vi "Float To String.vi"(4 "Type Enum [auto]":T1, 5 "Formatting (auto)":string, 6 "Variant":variant, 8 "error in (no error)":errorcluster, 10 "Multiply":variant, 11 "Registry Object":refnum<class "Carya Config.lvclass">) -> (0 "error out":errorcluster, 2 "resulting string":string, 3 "Registry Object":refnum<class "Carya Config.lvclass">)   [LabVIEW 2013, in "Carya Config.lvclass"]
doc: "Copyright 2018, Carya Automatisering, Wiebe Walstra."
uses:
  Carya Config.lvclass
  <vilib>/Utility/VariantDataType/Type.ctl
  <vilib>/Utility/error.llb/Error Cluster From Error Code.vi
  <vilib>/ErrorRing/Error Ring.xnode
  CConfig Variant Accessor/CConfig Variant Accessor.lvclass
  <vilib>/Utility/VariantDataType/VariantType.lvlib
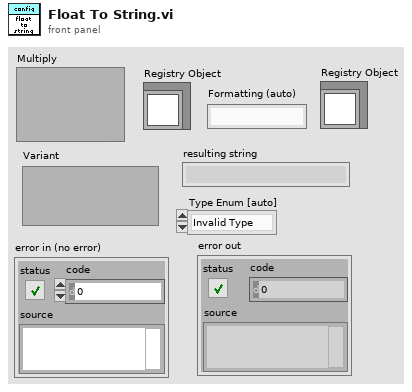
[diagram p1: front panel]
types:
  T1 = typedef "VariantType.lvlib/Type.ctl" = enum8{"Invalid Type", "Void", "I8", "I16", "I32", "I64", "U8", "U16", "U32", "U64", "Single Float", "Double Float", "Extended Float", "Single Complex", "Double Complex", "Extended Complex", "Enum U8", "Enum U16", "Enum U32", "Enum U64", "Single Float With Unit", "Double Float With Unit", "Extended Float With Unit", "Single Complex with Unit", "Double Complex with Unit", "Extended Complex with Unit", "Boolean", "String", "Path", "Picture", "Tag", "Array", "Cluster", "Variant", "LV Variant", "Waveform", "Timestamp", "Digital Waveform", "Digital Data", "ExpressData", "Refnum", "External Data", "VI", "Poly VI", "LabVIEW Class Instance", "Fixed Point"}
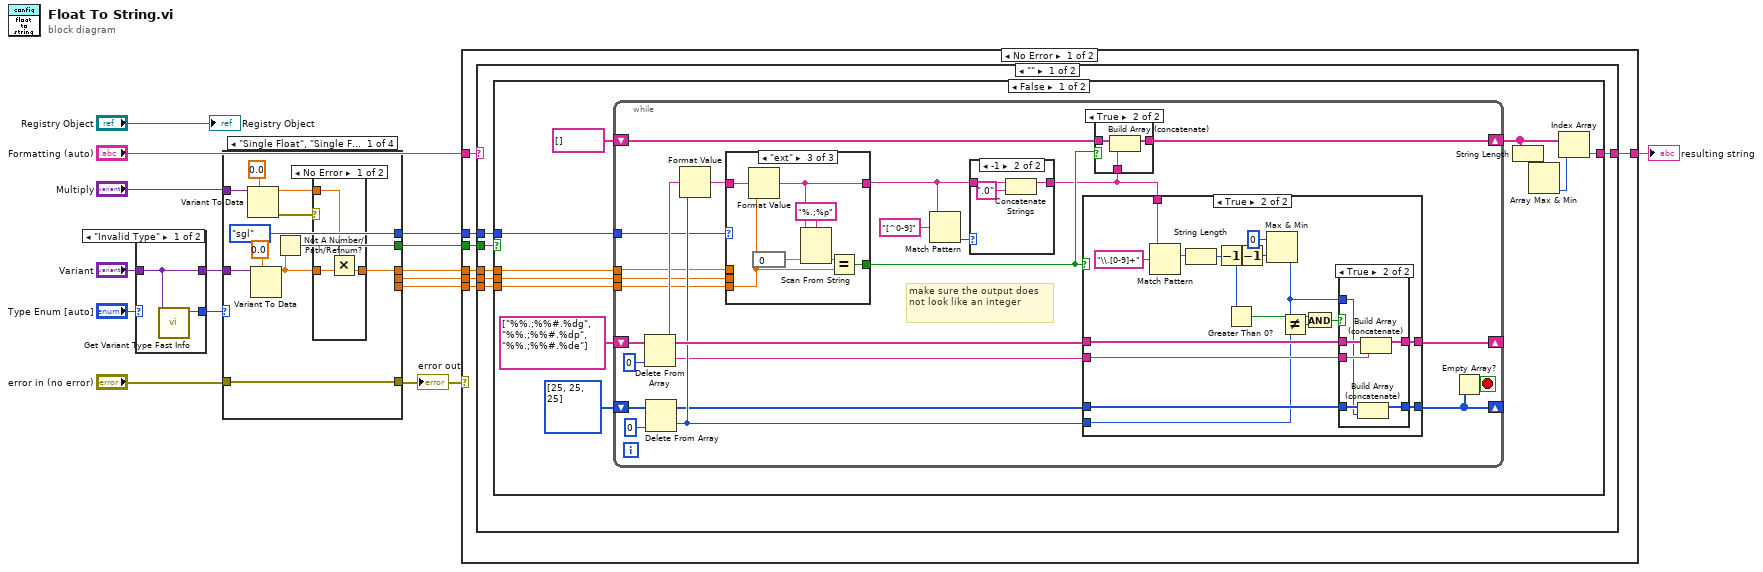
[diagram p0: block diagram]
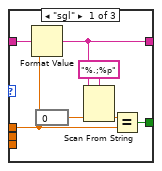
[diagram p3: hidden frame]
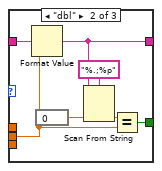
[diagram p4: hidden frame]
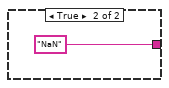
[diagram p8: hidden frame]
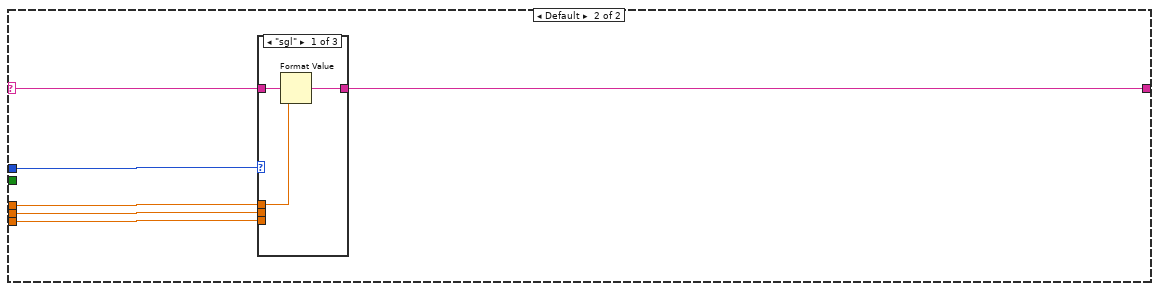
[diagram p9: hidden frame]
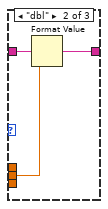
[diagram p10: hidden frame]
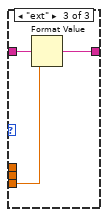
[diagram p11: hidden frame]
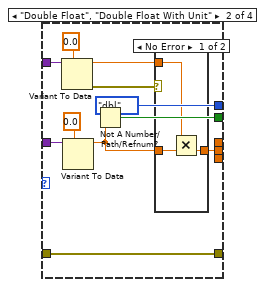
[diagram p15: hidden frame]
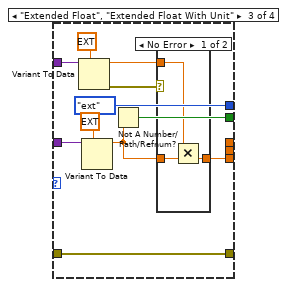
[diagram p17: hidden frame]
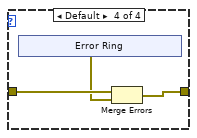
[diagram p19: hidden frame]
diagram:
  n1 = case shown="\"Invalid Type\"" "Type Enum [auto]" {
    selector: "Type Enum [auto]" -> [_ w19]
    tunnel: "Variant" -> [w16 w18]
    tunnel: [w17 w19] -> w5
    tunnel: [w16 w18] -> w7
    frame "Invalid Type" {
      n2 = call "Get Variant Type Fast Info.vi"("Variant"=w16) -> ("Type Enum"=w17:T1)  [unwired: 6 in, 4 out]
    }
    frame Default {
    }
  }
  n3 = case shown="\"Single Float\", \"Single Float With Unit\"" w5 {
    tunnel: [w22 _ _ _] -> w1
    tunnel: [w30 w45 w60 _] -> w13
    tunnel: [_ _ w50 _] -> w12
    tunnel: [_ w35 _ _] -> w11
    tunnel: w7 -> [w28 w43 w58 _]
    tunnel: [enum16{"sgl", "dbl", "ext"}."sgl" ("Type [dbl]") enum16{"sgl", "dbl", "ext"}."dbl" ("Type [dbl]") enum16{"sgl", "dbl", "ext"}."ext" ("Type [dbl]") _] -> w6
    tunnel: "error in (no error)" -> [w26 w41 w56 w67]
    tunnel: [w26 w41 w56 w65] -> w3
    tunnel: "Multiply" -> [w24 w39 w54 _]
    frame "Single Float", "Single Float With Unit" {
      n4 = Variant To Data(type=sgl 0.0, Variant=w24) -> (data=w21:sgl, error out=w20:errorcluster)  [unwired: 1 in]
      n5 = Variant To Data(type=sgl 0.0, Variant=w28) -> (data=w23:sgl)  [unwired: 1 in, 1 out]
      n6 = Not A Number/Path/Refnum?(number/path/refnum=w23) -> (NaN/Path/Refnum?=w30:bool)
      n7 = case shown="No Error" w20 {
        tunnel: w23 -> [w33 w34]
        tunnel: [w32 w34] -> w22
        tunnel: w21 -> [w31 _]
        frame No Error {
          n8 = Multiply(x=w31, y=w33) -> (x*y=w32:sgl)
        }
        frame Error {
        }
      }
    }
    frame "Double Float", "Double Float With Unit" {
      n9 = Variant To Data(type=0.0, Variant=w39) -> (data=w37:dbl, error out=w38:errorcluster)  [unwired: 1 in]
      n10 = Variant To Data(type=0.0, Variant=w43) -> (data=w36:dbl)  [unwired: 1 in, 1 out]
      n11 = Not A Number/Path/Refnum?(number/path/refnum=w36) -> (NaN/Path/Refnum?=w45:bool)
      n12 = case shown="No Error" w38 {
        tunnel: w36 -> [w48 w49]
        tunnel: [w47 w49] -> w35
        tunnel: w37 -> [w46 _]
        frame No Error {
          n13 = Multiply(x=w46, y=w48) -> (x*y=w47:dbl)
        }
        frame Error {
        }
      }
    }
    frame "Extended Float", "Extended Float With Unit" {
      n14 = Variant To Data(type=ext 0.0, Variant=w54) -> (data=w53:ext, error out=w52:errorcluster)  [unwired: 1 in]
      n15 = Variant To Data(type=ext 0.0, Variant=w58) -> (data=w51:ext)  [unwired: 1 in, 1 out]
      n16 = Not A Number/Path/Refnum?(number/path/refnum=w51) -> (NaN/Path/Refnum?=w60:bool)
      n17 = case shown="No Error" w52 {
        tunnel: w51 -> [w63 w64]
        tunnel: [w62 w64] -> w50
        tunnel: w53 -> [w61 _]
        frame No Error {
          n18 = Multiply(x=w61, y=w63) -> (x*y=w62:ext)
        }
        frame Error {
        }
      }
    }
    frame Default {
      n19 = xnode "Error Ring"() -> ("error out"=w66:errorcluster)
      n20 = Merge Errors(w67, w66) -> (w65:errorcluster)
    }
  }
  "error out" <- w3
  n21 = case shown="No Error" w3 {
    tunnel: [w79 _] -> w15
    tunnel: w1 -> [w78 _]
    tunnel: w13 -> [w77 _]
    tunnel: w12 -> [w76 _]
    tunnel: w11 -> [w75 _]
    tunnel: "Formatting (auto)" -> [w74 _]
    tunnel: w6 -> [w73 _]
    frame No Error {
      n22 = case shown="\"\"" w74 {
        selector: w74 -> [_ w178]
        tunnel: [w85 w177] -> w79
        tunnel: w78 -> [w84 w182]
        tunnel: w77 -> [w83 _]
        tunnel: w76 -> [w82 w181]
        tunnel: w75 -> [w81 w180]
        tunnel: w73 -> [w80 w179]
        frame "" {
          n23 = case shown="False" w83 {
            tunnel: [w94 "NaN" ("output string")] -> w85
            tunnel: w84 -> [w90 _]
            tunnel: w82 -> [w88 _]
            tunnel: w81 -> [w87 _]
            tunnel: w80 -> [w86 _]
            frame False {
              n24 = while {
                tunnel: w90 -> [w104]
                shift-right: [w117] -> w92
                shift-left: string[] [] -> [w118]
                shift-right: [w109] -> _
                shift-left: string[] ["%%.;%%#.%dg", "%%.;%%#.%dp", "%%.;%%#.%de"] -> [w116]
                shift-right: [w106] -> _
                shift-left: i32[] [25, 25, 25] -> [w115]
                tunnel: w88 -> [w102]
                tunnel: w87 -> [w103]
                tunnel: w86 -> [w101]
                stop <- w105 stop-if-true
                # "make sure the output does not look like an integer"
                n25 = Delete From Array(array=w116, index=0) -> (deleted portion=w108:string, array with subset deleted=w111:string[])  [unwired: 1 in]
                n26 = Delete From Array(array=w115, index=0) -> (deleted portion=w110:i32, array with subset deleted=w107:i32[])  [unwired: 1 in]
                n27 = Format Value(format string=w108, value (0)=w110) -> (output string=w119:string)  [unwired: 1 in]
                n28 = case shown="\"ext\"" w101 {
                  tunnel: w119 -> [w130 w137 w144]
                  tunnel: [w129 w136 w143] -> w112
                  tunnel: [w128 w135 w142] -> w97
                  tunnel: w104 -> [w127 _ _]
                  tunnel: w103 -> [_ w131 _]
                  tunnel: w102 -> [_ _ w138]
                  frame "sgl" {
                    n29 = Format Value(format string=w130, value (0)=w127) -> (output string=w128:string)  [unwired: 1 in]
                    n30 = expression code="0"(w127) -> (w124:sgl)
                    n31 = Scan From String(format string="%.;%p", input string=w128, default 1=w124) -> (output 1=w125:sgl)  [unwired: 2 in, 3 out]
                    n32 = Equal?(x=w125, y=w127) -> (x = y?=w129:bool)
                  }
                  frame "dbl" {
                    n33 = Format Value(format string=w137, value (0)=w131) -> (output string=w135:string)  [unwired: 1 in]
                    n34 = expression code="0"(w131) -> (w132:dbl)
                    n35 = Scan From String(format string="%.;%p", input string=w135, default 1=w132) -> (output 1=w133:dbl)  [unwired: 2 in, 3 out]
                    n36 = Equal?(x=w133, y=w131) -> (x = y?=w136:bool)
                  }
                  frame "ext" {
                    n37 = Format Value(format string=w144, value (0)=w138) -> (output string=w142:string)  [unwired: 1 in]
                    n38 = expression code="0"(w138) -> (w139:ext)
                    n39 = Scan From String(format string="%.;%p", input string=w142, default 1=w139) -> (output 1=w140:ext)  [unwired: 2 in, 3 out]
                    n40 = Equal?(x=w140, y=w138) -> (x = y?=w143:bool)
                  }
                }
                n41 = Match Pattern(string=w97, regular expression="[^0-9]") -> (offset past match=w99:i32)  [unwired: 1 in, 3 out]
                n42 = case shown="-1" w99 {
                  tunnel: [w120 w122] -> w98
                  tunnel: w97 -> [w120 w123]
                  frame Default {
                  }
                  frame -1 {
                    n43 = Concatenate Strings(w123, ".0" ("string")) -> (w122:string)
                  }
                }
                n44 = case shown="True" w112 {
                  tunnel: w111 -> [w146 w157]
                  tunnel: w98 -> [_ w161]
                  tunnel: w110 -> [_ w153]
                  tunnel: [w146 w156] -> w109
                  tunnel: w108 -> [_ w155]
                  tunnel: w107 -> [w145 w154]
                  tunnel: [w145 w152] -> w106
                  frame False {
                  }
                  frame True {
                    n45 = Match Pattern(string=w161, regular expression="\\.[0-9]+") -> (match substring=w163:string)  [unwired: 1 in, 3 out]
                    n46 = String Length(string=w163) -> (length=w150:i32)
                    n47 = Decrement(x=w150) -> (x-1=w148:i32)
                    n48 = Greater Than 0?(x=w148) -> (x > 0?=w149:bool)
                    n49 = Decrement(x=w148) -> (x-1=w160:i32)
                    n50 = Max & Min(x=0, y=w160) -> (max(x,y)=w147:i32)  [unwired: 1 out]
                    n51 = Not Equal?(x=w147, y=w153) -> (x != y?=w158:bool)
                    n52 = And(x=w149, y=w158) -> (x .and. y?=w151:bool)
                    n53 = case shown="True" w151 {
                      tunnel: w157 -> [w165 w171]
                      tunnel: [w165 w170] -> w156
                      tunnel: w155 -> [_ w169]
                      tunnel: w154 -> [w164 w168]
                      tunnel: w147 -> [_ w167]
                      tunnel: [w164 w166] -> w152
                      frame False {
                      }
                      frame True {
                        n54 = Build Array (concatenate)(w168, w167) -> (w166:i32[])
                        n55 = Build Array (concatenate)(w171, w169) -> (w170:string[])
                      }
                    }
                  }
                }
                n56 = case shown="True" w112 {
                  tunnel: w118 -> [w172 w175]
                  tunnel: [w172 w174] -> w117
                  tunnel: w98 -> [_ w173]
                  frame False {
                  }
                  frame True {
                    n57 = Build Array (concatenate)(w175, w173) -> (w174:string[])
                  }
                }
                n58 = Empty Array?(array=w106) -> (empty?=w105:bool)
              }
              n59 = String Length(string=w92) -> (length=w96:i32[])
              n60 = Array Max & Min(array=w96) -> (min index (indices)=w95:i32)  [unwired: 3 out]
              n61 = Index Array(array=w92, index=w95) -> (element=w94:string)
            }
            frame True {
            }
          }
        }
        frame Default {
          n62 = case shown="\"sgl\"" w179 {
            tunnel: w178 -> [w185 w188 w191]
            tunnel: [w184 w187 w190] -> w177
            tunnel: w182 -> [w183 _ _]
            tunnel: w180 -> [_ w186 _]
            tunnel: w181 -> [_ _ w189]
            frame "sgl" {
              n63 = Format Value(format string=w185, value (0)=w183) -> (output string=w184:string)  [unwired: 1 in]
            }
            frame "dbl" {
              n64 = Format Value(format string=w188, value (0)=w186) -> (output string=w187:string)  [unwired: 1 in]
            }
            frame "ext" {
              n65 = Format Value(format string=w191, value (0)=w189) -> (output string=w190:string)  [unwired: 1 in]
            }
          }
        }
      }
    }
    frame Error {
    }
  }
  "resulting string" <- w15
  "Registry Object" <- "Registry Object"
